vi "Fetch Measurements.vi"(0 "VISA resource name":refnum<visa-resource-name>, 5 "Timeout (10000 ms)":i32=10000 format="%#.6g", 11 "error in (no error)":errorcluster) -> (3 "Voltage":sgl[](array[numeric]), 4 "VISA resource name out":refnum<visa-resource-name>, 6 "Current":sgl[](array[numeric]), 8 "Resistance":sgl[](array[numeric]), 10 "Timestamp":sgl[](array[numeric]), 14 "Status":sgl[](array[numeric]), 15 "error out":errorcluster)   [LabVIEW 2010]
doc: "Fetches data for voltage, current, resistance, timestamp, and status. These readings are then provided in separate arrays for each type of reading.\n\n<B>Note</B> Use this VI only with other low-level VIs. The high-level VIs automatically incorporate this functionality. This VI does not check the instrument status. If you want to check the instrument status, call the Error Query VI at the conclusion of the sequence."
panel:
  out "return count":u32
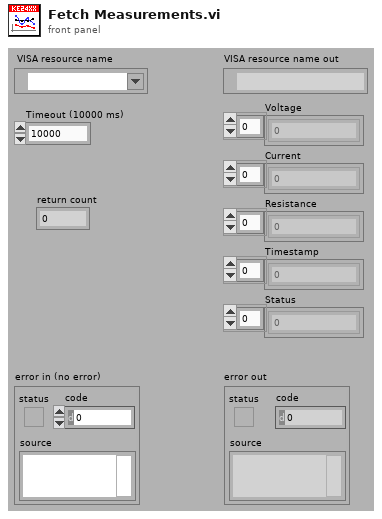
[diagram p1: front panel]
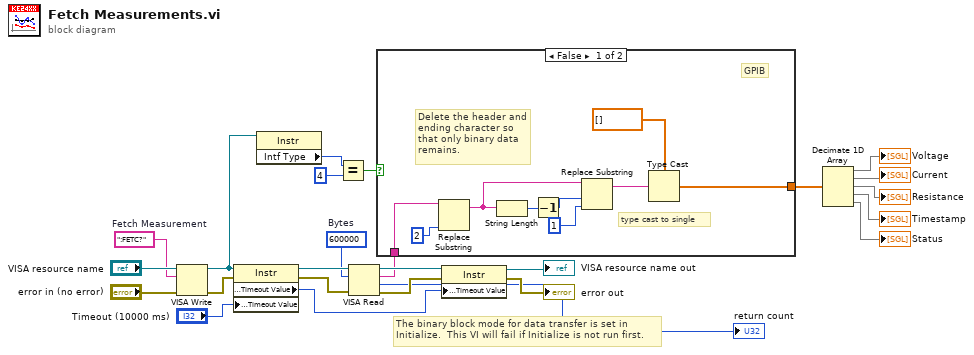
[diagram p0: block diagram]
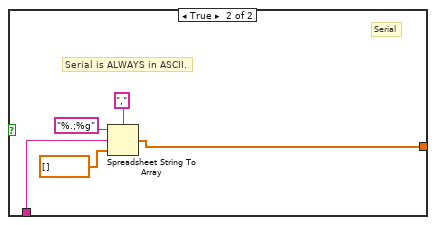
[diagram p2: hidden frame]
diagram:
  w23 = ":FETC?"  # Fetch Measurement
  w13 = u32 600000  # Bytes
  # "The binary block mode for data transfer is set in Initialize.  This VI will fail if Initialize is not run first."
  n1 = VISA Write(VISA resource name="VISA resource name", write buffer=w23, error in (no error)="error in (no error)") -> (VISA resource name out=w5:refnum<visa-resource-name>, error out=w22:errorcluster)  [unwired: 1 out]
  n2 = property class="Instr"(reference=w5, error in=w22, "General Settings:Timeout Value"="Timeout (10000 ms)") -> (reference out=w21:refnum<visa-resource-name>, error out=w20:errorcluster, "General Settings:Timeout Value"=w16:u32)
  n3 = property class="Instr"(reference=w5) -> ("Intf Type"=w4:u16)  [unwired: 1 in, 2 out]
  n4 = Equal?(x=w4, y=u16 4) -> (x = y?=w2:bool)
  n5 = VISA Read(VISA resource name=w21, byte count=w13, error in (no error)=w20) -> (VISA resource name out=w18:refnum<visa-resource-name>, read buffer=w12:string, return count=→"return count":u32, error out=w17:errorcluster)
  n6 = case shown="False" w2 {
    tunnel: w12 -> [w34 w39]
    tunnel: [w26 w35] -> w11
    frame False {
      # "Delete the header and ending character so that only binary data remains."
      # "GPIB"
      # "type cast to single"
      n7 = Replace Substring(2:2 ("length (len. of substring)"), 5:w34) -> (1:w32:string)  [unwired: 2 in, 1 out]
      n8 = String Length(string=w32) -> (length=w31:i32)
      n9 = Decrement(x=w31) -> (x-1=w30:i32)
      n10 = Replace Substring(2:1 ("length (len. of substring)"), 3:w30, 5:w32) -> (1:w28:string)  [unwired: 1 in, 1 out]
      n11 = Type Cast(type=sgl[] [], x=w28) -> (*(type *) &x=w26:sgl[])
    }
    frame True {
      # "Serial is ALWAYS in ASCII."
      # "Serial"
      n12 = Spreadsheet String To Array(delimiter (Tab)=",", format string="%.;%g", spreadsheet string=w39, array type (2D Dbl)=sgl[] []) -> (array=w35:sgl[])
    }
  }
  n13 = property class="Instr"(reference=w18, error in=w17, "General Settings:Timeout Value"=w16) -> (reference out=→"VISA resource name out":refnum<visa-resource-name>, error out=→"error out":errorcluster)
  n14 = Decimate 1D Array(w11) -> (→"Voltage":sgl[], →"Current":sgl[], →"Resistance":sgl[], →"Timestamp":sgl[], →"Status":sgl[])
